vi "Initialize KH Cluster.vi"(8 "error in (no error)":errorcluster, 10 "KH Addresses":refnum<visa-resource-name>[](array[refnum]) caption="KH Address[A,B,C,...]") -> (0 "error out":errorcluster, 3 "KH Cluster out":T1)   [LabVIEW 2016, in "Control Experiment UI.lvclass"]
uses:
  Control Experiment UI.lvclass
  Typedefs/KH Cluster--Cluster.ctl
  <userlib>/LevyLab/Krohn Hite 7008/typedefs/SetAll-Cluster.ctl
  <userlib>/LevyLab/Krohn Hite 7008/typedefs/Channel-Enum.ctl
  <userlib>/LevyLab/Krohn Hite 7008/typedefs/Gain-Enum.ctl
  <userlib>/LevyLab/Krohn Hite 7008/typedefs/Filter-Enum.ctl
  <userlib>/LevyLab/Krohn Hite 7008/typedefs/Shunt-Enum.ctl
  <userlib>/LevyLab/Krohn Hite 7008/typedefs/Coupling-Enum.ctl
  <userlib>/LevyLab/Krohn Hite 7008/typedefs/Input Configuration-Enum.ctl
  <userlib>/LevyLab/Krohn Hite 7008/Instrument.KH7008.lvclass
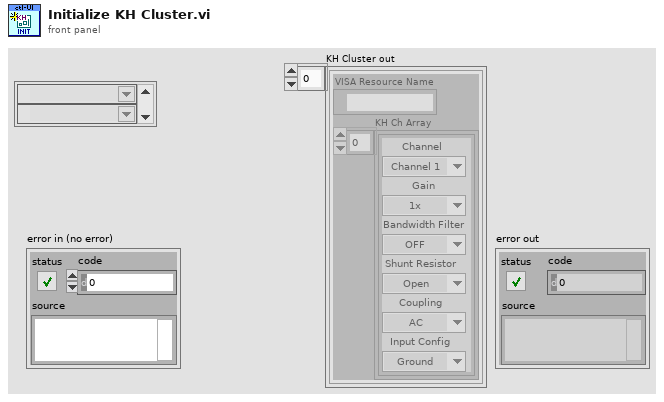
[diagram p1: front panel]
types:
  T1 = typedef "KH Cluster--Cluster.ctl" = cluster{"VISA Resource Name":refnum<visa-resource-name>, "KH Ch Array":T2[]}[]
  T2 = typedef "Instrument.KH7008.lvclass/SetAll-Cluster.ctl" = cluster{"Channel":T3, "Gain":T4, "Bandwidth Filter":T5, "Shunt Resistor":T6, "Coupling":T7, "Input Config":T8}
  T3 = typedef "Instrument.KH7008.lvclass/Channel-Enum.ctl" = enum16{"Channel 1", "Channel 2", "Channel 3", "Channel 4", "Channel 5", "Channel 6", "Channel 7", "Channel 8"}
  T4 = typedef "Instrument.KH7008.lvclass/Gain-Enum.ctl" = enum16{"1x", "10x", "100x", "1000x"}
  T5 = typedef "Instrument.KH7008.lvclass/Filter-Enum.ctl" = enum16{"OFF", "ON"}
  T6 = typedef "Instrument.KH7008.lvclass/Shunt-Enum.ctl" = enum16{"Open", "50 Ohms", "500 Ohms", "5k Ohms", "50k Ohms", "10M Ohm"}
  T7 = typedef "Instrument.KH7008.lvclass/Coupling-Enum.ctl" = enum16{"AC", "DC"}
  T8 = typedef "Instrument.KH7008.lvclass/Input Configuration-Enum.ctl" = enum16{"Ground", "SE+ (-gnd)", "SE- (+gnd)", "Differential"}
  T9 = cluster{"VISA Resource Name":refnum<visa-resource-name>, T2[]}
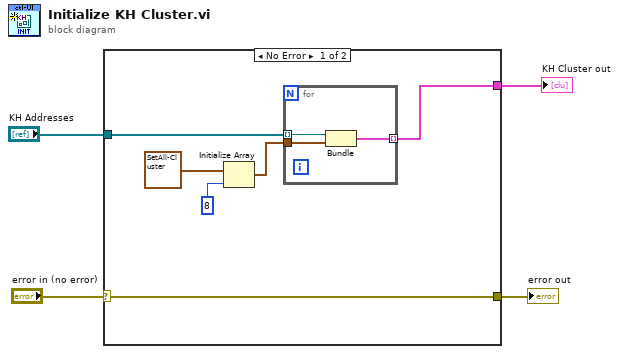
[diagram p0: block diagram]
diagram:
  n1 = case shown="No Error" "error in (no error)" {
    selector: "error in (no error)" -> [w6 w14]
    tunnel: "KH Addresses" -> [w9 _]
    tunnel: [w7 _] -> w3
    tunnel: [w6 w14] -> w1
    frame No Error {
      n2 = Initialize Array(T2 {"Channel"=enum."Channel 1", "Gain"=enum."10x", "Bandwidth Filter"=enum."ON", "Shunt Resistor"=enum."50 Ohms", "Coupling"=enum."DC", "Input Config"=enum."Differential"} ("Channel Settings"), 8 ("dimension size")) -> (w8:T2[])
      n3 = for {
        tunnel: w9 -> [w13] mode=indexing
        tunnel: w8 -> [w12]
        tunnel: [w11] -> w7 mode=indexing
        n4 = Bundle("VISA Resource Name"=w13, w12) -> (w11:T9)  [unwired: 1 in]
      }
    }
    frame Error {
    }
  }
  "KH Cluster out" <- w3
  "error out" <- w1
